vi "EM CCD Gain  - subvi.vi"(8 "error in (no error)":errorcluster, 11 "EM CCD Gain":u16) -> (0 "error out":errorcluster)   [LabVIEW 2014]
uses:
  Library Files - Andor and MadCity/Andorlib/atmcd32d.lvlib
panel:
  out "function return":u32
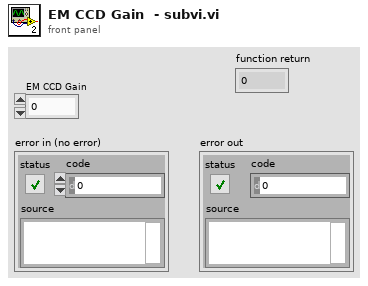
[diagram p1: front panel]
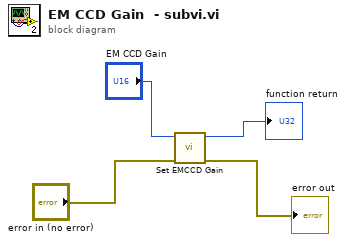
[diagram p0: block diagram]
diagram:
  n1 = call "Set EMCCD Gain.vi"("error in (no error)"="error in (no error)", "gain"="EM CCD Gain") -> ("error out"=→"error out":errorcluster, "function return"=→"function return":u32)  [unwired: 8 in]
